vi "Internal Servomech Gyro Set Position.vi"(0 "TurretDevRef":T1={"MotorControlDevRef"={"DeviceStatus"={"status"=FALSE, "code"=0, "source"=""}, "Type"=enum."PWM", "PWM"={"Digital Module"=enum."Digital Module 1", "PWM Channel"=enum."Invalid", "DeadBand"={"Name"="", "maxPositivePwm"=0, "minPositivePwm"=0, "centerPwm"=0, "maxNegativePwm"=0, "minNegativePwm"=0, "angularRange"=0}}, "CAN"={"Device Number"=0, "Control Mode"=enum."Percent VBus", "Semaphore"=refnum, "Max Vout"=12.0}, "Invert"=FALSE, "TransformRef"=refnum, "InvTransformRef"=refnum}, "LauncherGyro"={"DevStatus"={"status"=FALSE, "code"=0, "source"=""}, "Analog Module"=enum."Analog Module 1", "Analog Channel"=enum."AI 1", "Offset"=0.0, "Gain (VoltsPerDegree/Second)"=0.0}, "RobotGyro"={"DevStatus"={"status"=FALSE, "code"=0, "source"=""}, "Analog Module"=enum."Analog Module 1", "Analog Channel"=enum."AI 1", "Offset"=0.0, "Gain (VoltsPerDegree/Second)"=0.0}, "Difference Range"={"Max Difference"=0.0, "Min Difference"=0.0}, "Dead Band Tolerance"=0.0}, 1 "PID gains":T12={"proportional gain (Kc)"=1.0, "integral time (Ti, min)"=0.01, "derivative time (Td, min)"=0.0} {"derivative time (Td, min)" format="%.3f"; "integral time (Ti, min)" format="%.3f"; "proportional gain (Kc)" format="%.3f"}, 5 "Desired Gyro position":dbl format="%.2f", 11 "error in":errorcluster, 12 "reinitialize? (F)":bool, 14 "Use dead band?":bool) -> (4 "TurretDevRef":T1={"MotorControlDevRef"={"DeviceStatus"={"status"=FALSE, "code"=0, "source"=""}, "Type"=enum."PWM", "PWM"={"Digital Module"=enum."Digital Module 1", "PWM Channel"=enum."Invalid", "DeadBand"={"Name"="", "maxPositivePwm"=0, "minPositivePwm"=0, "centerPwm"=0, "maxNegativePwm"=0, "minNegativePwm"=0, "angularRange"=0}}, "CAN"={"Device Number"=0, "Control Mode"=enum."Percent VBus", "Semaphore"=refnum, "Max Vout"=12.0}, "Invert"=FALSE, "TransformRef"=refnum, "InvTransformRef"=refnum}, "LauncherGyro"={"DevStatus"={"status"=FALSE, "code"=0, "source"=""}, "Analog Module"=enum."Analog Module 1", "Analog Channel"=enum."AI 1", "Offset"=0.0, "Gain (VoltsPerDegree/Second)"=0.0}, "RobotGyro"={"DevStatus"={"status"=FALSE, "code"=0, "source"=""}, "Analog Module"=enum."Analog Module 1", "Analog Channel"=enum."AI 1", "Offset"=0.0, "Gain (VoltsPerDegree/Second)"=0.0}, "Difference Range"={"Max Difference"=0.0, "Min Difference"=0.0}, "Dead Band Tolerance"=0.0}, 6 "Error":dbl, 8 "Hit dead band?":bool, 10 "In Range?":bool, 15 "error out":errorcluster)   [LabVIEW 2011]
uses:
  TurretDevRef.ctl
  <vilib>/Rock Robotics/WPI/MotorControl/WPI_MotorControlDeviceRef.ctl
  <vilib>/Rock Robotics/SystemInterfaces/Typedef/FPGA_TypedefDigitalModule.ctl
  <vilib>/Rock Robotics/SystemInterfaces/DIO/FPGA_DIOPWMChannel.ctl
  <vilib>/Rock Robotics/WPI/PWM/WPI_PWMDeadband.ctl
  <vilib>/Rock Robotics/WPI/CAN/Jaguar/SubVIs/WPI_CANJaguar_ControlMode.ctl
  <vilib>/Rock Robotics/WPI/PWM/WPI_PWMTransform_ConPane.ctl
  <vilib>/Rock Robotics/WPI/Gyro/WPI_GyroDevRef.ctl
  <vilib>/Rock Robotics/SystemInterfaces/Typedef/FPGA_TypedefAnalogModule.ctl
  <vilib>/Rock Robotics/SystemInterfaces/AI/FPGA_AIChannel.ctl
  <vilib>/addons/control/pid/pid.llb/PID (DBL).vi
  <vilib>/addons/control/pid/NI_PID_pid.lvlib
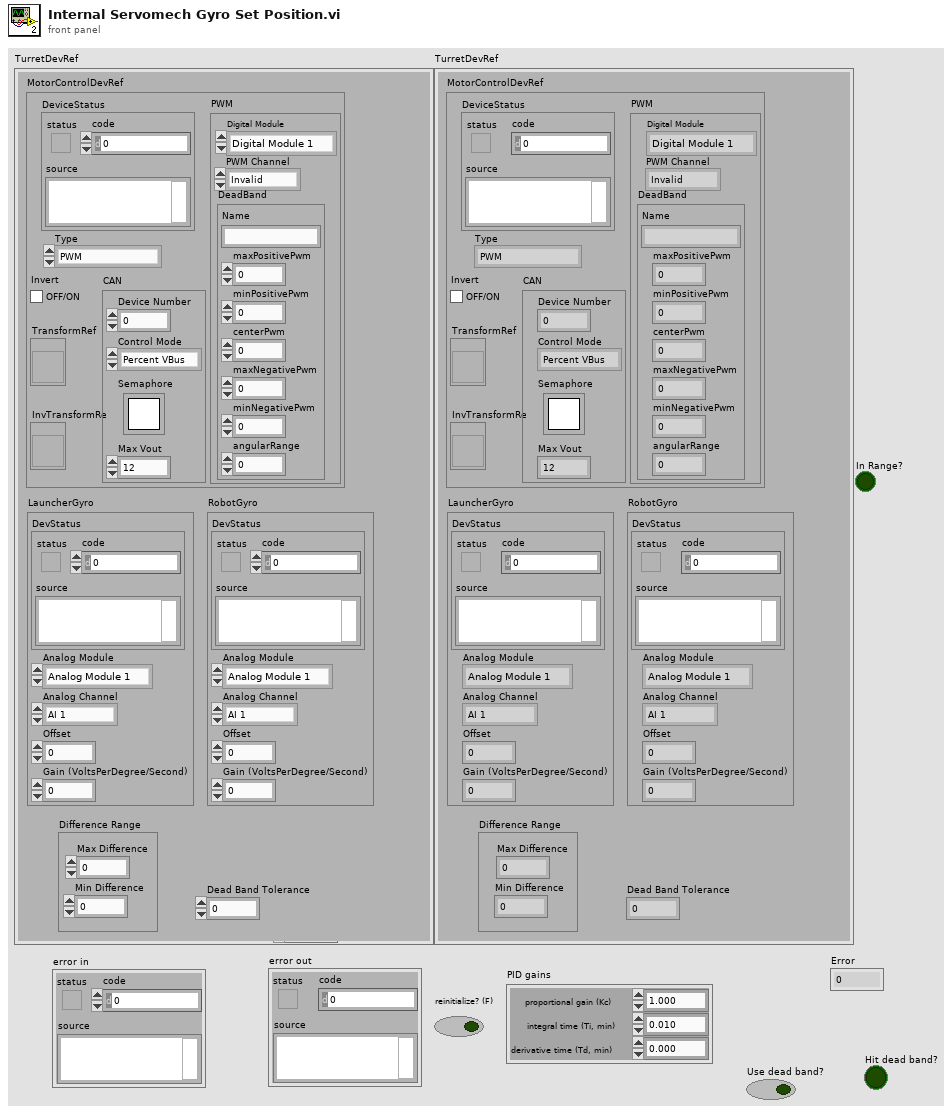
[diagram p1: front panel]
types:
  T1 = typedef "TurretDevRef.ctl" = cluster{"MotorControlDevRef":T2, "LauncherGyro":T9, "RobotGyro":T9, "Difference Range":cluster{"Max Difference":dbl, "Min Difference":dbl}, "Dead Band Tolerance":dbl}
  T2 = typedef "WPI_MotorControlDeviceRef.ctl" = cluster{"DeviceStatus":errorcluster, "Type":enum16{"PWM", "CAN"}, "PWM":cluster{"Digital Module":T3, "PWM Channel":T4, "DeadBand":T5}, "CAN":cluster{"Device Number":u8, "Control Mode":T6, "Semaphore":T7, "Max Vout":dbl}, "Invert":bool, "TransformRef":T8, "InvTransformRef":T8}
  T3 = typedef "FPGA_TypedefDigitalModule.ctl" = enum16{"Digital Module 1", "Digital Module 2"}
  T4 = typedef "FPGA_DIOPWMChannel.ctl" = enum8{"PWM 1", "PWM 2", "PWM 3", "PWM 4", "PWM 5", "PWM 6", "PWM 7", "PWM 8", "PWM 9", "PWM 10", "Invalid"}
  T5 = typedef "WPI_PWMDeadband.ctl" = cluster{"Name":string, "maxPositivePwm":i32, "minPositivePwm":i32, "centerPwm":i32, "maxNegativePwm":i32, "minNegativePwm":i32, "angularRange":u16}
  T6 = typedef "WPI_CANJaguar_ControlMode.ctl" = enum8{"Percent VBus", "Current", "Speed", "Position", "Voltage"}
  T7 = typedef "Semaphore RefNum" = refnum<k1>
  T8 = typedef "WPI_PWMTransform_ConPane.ctl" = refnum<vi>
  T9 = typedef "WPI_GyroDevRef.ctl" = cluster{"DevStatus":errorcluster, "Analog Module":T10, "Analog Channel":T11, "Offset":dbl, "Gain (VoltsPerDegree/Second)":dbl}
  T10 = typedef "FPGA_TypedefAnalogModule.ctl" = enum16{"Analog Module 1", "Analog Module 2"}
  T11 = typedef "FPGA_AIChannel.ctl" = enum8{"AI 1", "AI 2", "AI 3", "AI 4", "AI 5", "AI 6", "AI 7", "AI 8", "Invalid"}
  T12 = cluster{"proportional gain (Kc)":dbl, "integral time (Ti, min)":dbl, "derivative time (Td, min)":dbl}
  T13 = cluster{"Max Difference":dbl, "Min Difference":dbl}
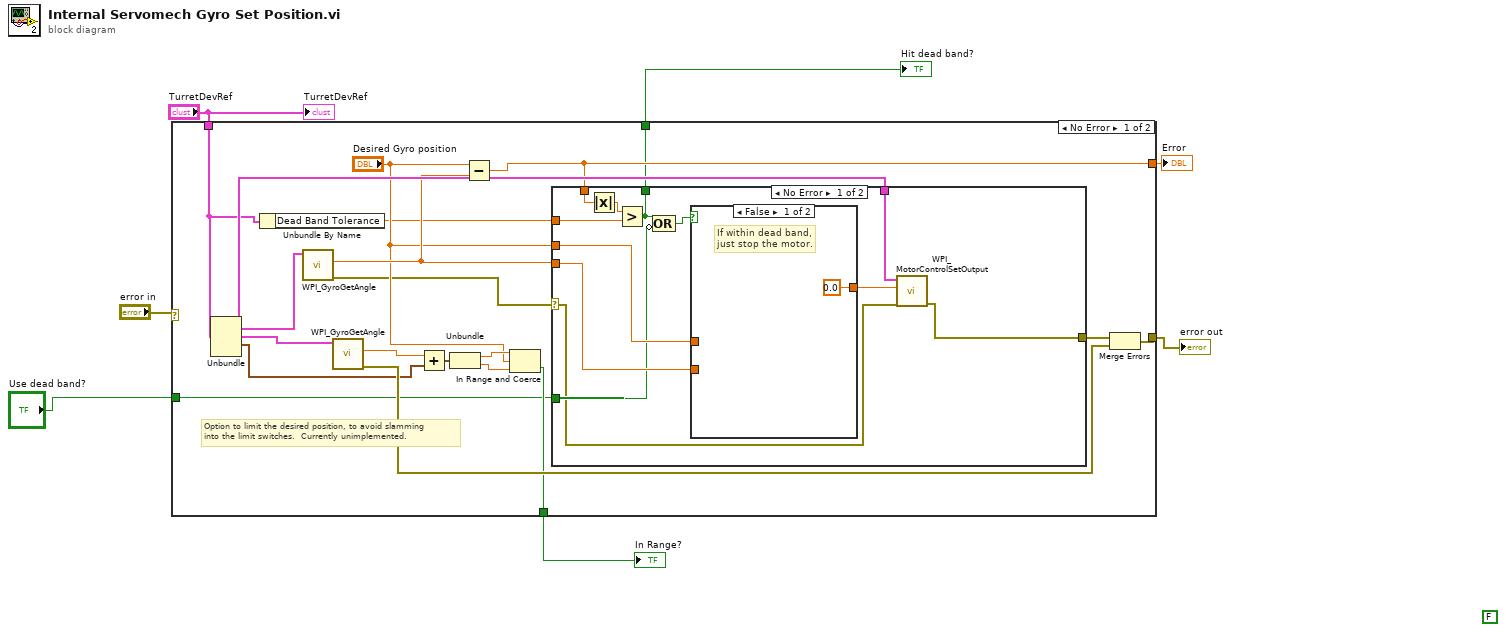
[diagram p0: block diagram]
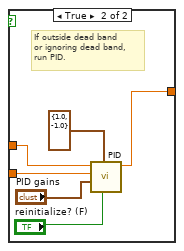
[diagram p2: hidden frame]
diagram:
  (unwired) FALSE
  n1 = case shown="No Error" "error in" {
    selector: "error in" -> [_ w48]
    tunnel: "TurretDevRef" -> [w12 _]
    tunnel: [w23 w48] -> w5
    tunnel: [w10 _] -> w4
    tunnel: [w14 _] -> w3
    tunnel: "Use dead band?" -> [w13 _]
    tunnel: [w8 _] -> w1
    frame No Error {
      # "Option to limit the desired position, to avoid slamming\ninto the limit switches.  Currently unimplemented."
      n2 = Unbundle(w12) -> ("MotorControlDevRef"=w25:T2, "LauncherGyro"=w27:T9, "RobotGyro"=w26:T9, "Difference Range"=w19:T13)  [unwired: 1 out]
      n3 = Unbundle By Name(w12) -> ("Dead Band Tolerance"=w9:dbl)
      n4 = call <vilib>:"WPI_GyroGetAngle.vi"("GyroDevRef"=w27) -> ("error out"=w11:errorcluster, "Angle"=w21:dbl)  [unwired: 7 in, 2 out]
      n5 = call <vilib>:"WPI_GyroGetAngle.vi"("GyroDevRef"=w26) -> ("error out"=w22:errorcluster, "Angle"=w20:dbl)  [unwired: 7 in, 2 out]
      n6 = Add(x=w20, y=w19) -> (x+y=w16:T13)
      n7 = Unbundle(w16) -> ("Max Difference"=w18:dbl, "Min Difference"=w17:dbl)
      n8 = Subtract(x="Desired Gyro position", y=w21) -> (x-y=w10:dbl)
      n9 = In Range and Coerce(upper limit=w18, x="Desired Gyro position", lower limit=w17) -> (In Range?=w14:bool)  [unwired: 1 out]
      n10 = case shown="No Error" w11 {
        selector: w11 -> [w34 w47]
        tunnel: w21 -> [w39 _]
        tunnel: "Desired Gyro position" -> [w38 _]
        tunnel: w25 -> [w33 _]
        tunnel: [w29 w47] -> w24
        tunnel: w13 -> [w30 _]
        tunnel: w10 -> [w35 _]
        tunnel: w9 -> [w36 _]
        tunnel: [w28 _] -> w8
        frame No Error {
          n11 = Absolute Value(x=w35) -> (abs(x)=w37:dbl)
          n12 = Greater?(x=w37, y=w36) -> (0:w28:bool)
          n13 = Compound Arithmetic op=OR(w28, invert w30) -> (w31:bool)
          n14 = case shown="False" w31 {
            tunnel: w39 -> [_ w46]
            tunnel: w38 -> [_ w45]
            tunnel: [0.0 ("output") w41] -> w32
            frame False {
              # "If within dead band,\njust stop the motor."
            }
            frame True {
              # "If outside dead band\nor ignoring dead band,\nrun PID."
              n15 = call-poly <vilib>:"PID.vi"("reinitialize? (F)"="reinitialize? (F)", "output range"=cluster{"output high":dbl, "output low":dbl} {"output high"=1.0, "output low"=-1.0}, "PID gains"="PID gains", "process variable"=w46, "setpoint"=w45) -> ("output"=w41:dbl)  [unwired: 5 in, 1 out]
            }
          }
          n16 = call <vilib>:"WPI_MotorControlSetOutput.vi"("error in (no error)"=w34, "Output"=w32, "MotorControlDevRef"=w33) -> ("error out"=w29:errorcluster)  [unwired: 7 in, 1 out]
        }
        frame Error {
        }
      }
      n17 = Merge Errors(w24, w22) -> (w23:errorcluster)
    }
    frame Error {
    }
  }
  "error out" <- w5
  "Error" <- w4
  "In Range?" <- w3
  "Hit dead band?" <- w1
  "TurretDevRef" <- "TurretDevRef"
